vi "Get Connected by index.vi"(8 "error in (no error)":errorcluster, 10 "index":i32, 11 "Motions in":refnum<class "Motions.lvclass">) -> (0 "error out":errorcluster, 2 "Connected":bool, 3 "Motions out":refnum<class "Motions.lvclass">)   [LabVIEW 2016, in "Hardware.lvlib" / "Motions.lvlib" / "Motions.lvclass"]
uses:
  <userlib>/Common Components/Hardware/Abstract System/Motions/Motions/Motions.lvclass
  <userlib>/Common Components/Hardware/Abstract System/Motions/Motions/Motions.lvclass/Motions.ctl
  <vilib>/Utility/error.llb/Error Cluster From Error Code.vi
  <vilib>/ErrorRing/Error Ring.xnode
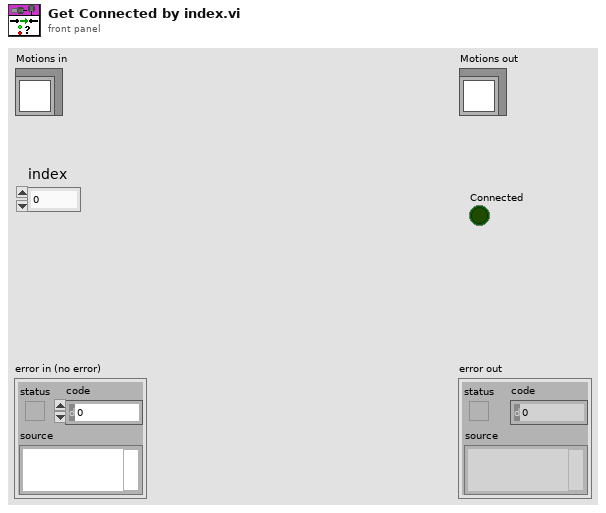
[diagram p1: front panel]
types:
  T1 = typedef "Hardware.lvlib/Motions.lvlib/Motions.lvclass/Motor States.ctl" = cluster{"Connected":bool, "Enabled":bool, "Moving Status":bool, "Soft Moving Status":bool, "Current Pos":dbl, "Target Pos":dbl, "Moving Dir (-1, 0, 1)":i32, "Error Status":bool, "Hard Limit+":bool, "Hard Limit-":bool, "Soft Limit+":bool, "Soft Limit-":bool, "History Dst Stack":refnum<queue>, "Motion Status":bool, "Motion TriggerAction Obj":refnum<class "TriggerAction Q.lvclass">}
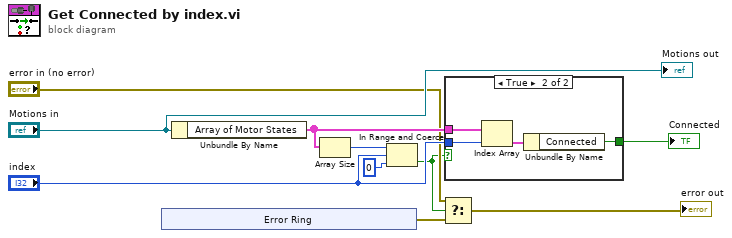
[diagram p0: block diagram]
diagram:
  n1 = xnode "Error Ring"() -> ("error out"=w3:errorcluster)
  n2 = Unbundle By Name("Motions in") -> ("Array of Motor States"=w8:T1[])
  n3 = Array Size(array=w8) -> (size(s)=w5:i32)
  n4 = In Range and Coerce(upper limit=w5, x="index", lower limit=0) -> (In Range?=w1:bool)  [unwired: 1 out]
  n5 = Select(t="error in (no error)", s=w1, f=w3) -> (s? t:f=→"error out":errorcluster)
  n6 = case shown="True" w1 {
    tunnel: [_ w13] -> w9
    tunnel: w8 -> [_ w12]
    tunnel: "index" -> [_ w11]
    frame False {
    }
    frame True {
      n7 = Index Array(array=w12, index=w11) -> (element=w14:T1)
      n8 = Unbundle By Name(w14) -> ("Connected"=w13:bool)
    }
  }
  "Connected" <- w9
  "Motions out" <- "Motions in"
